vi "clear the mutation history for the classes.vi"(11 "Path":path=path "D:/OneDrive - NI/_WorkingOn/CSM/Communicable-State-Machine/src/user.lib/_NEVSTOP/Communicable State Machine(CSM)/_Support/Priority Queue/Priority Queue.lvclass") -> ()   [LabVIEW 2017]
uses:
  <vilib>/Utility/EditLVLibs/LVClass/Mutation History.ctl
  <vilib>/Utility/EditLVLibs/LVClass/Mutation Record.ctl
  <vilib>/Utility/EditLVLibs/LibVersion.ctl
  <vilib>/Utility/EditLVLibs/Edit LVLibs.lvlib
panel:
  out "Mutation History":T1 {"LabVIEW Version" format="%.0x"}
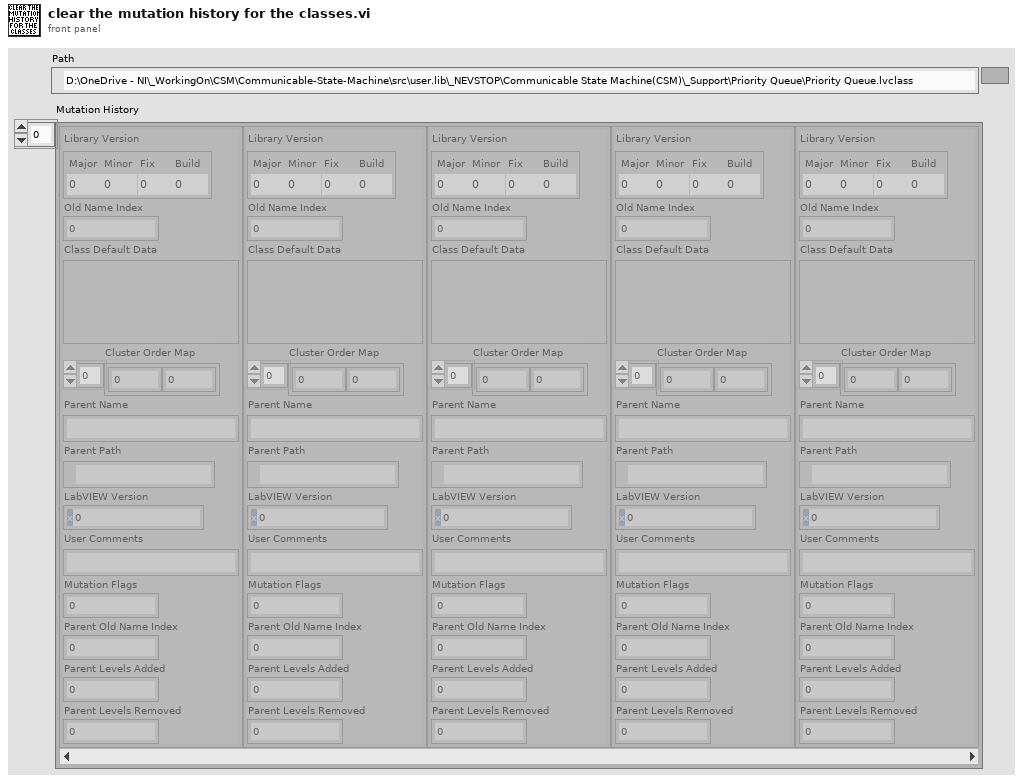
[diagram p1: front panel]
types:
  T1 = typedef "Edit LVLibs.lvlib/Mutation History.ctl" = T2[]
  T2 = typedef "Edit LVLibs.lvlib/Mutation Record.ctl" = cluster{"Library Version":T3, "Old Name Index":u8, "Class Default Data":variant, "Cluster Order Map":u32[], "Parent Name":string, "Parent Path":path, "LabVIEW Version":u32, "User Comments":string, "Mutation Flags":u8, "Parent Old Name Index":u8, "Parent Levels Added":u16, "Parent Levels Removed":u16}
  T3 = typedef "Edit LVLibs.lvlib/LibVersion.ctl" = cluster{"Major":u16, "Minor":u16, "Fix":u16, "Build":u16}
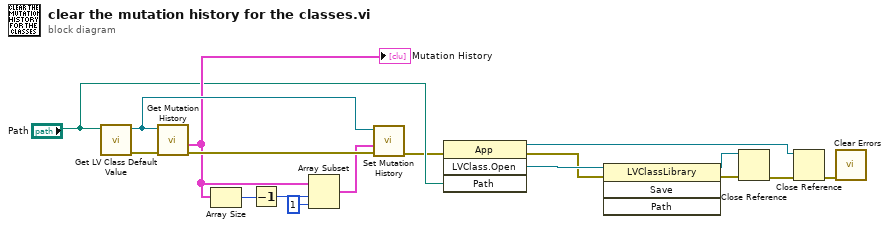
[diagram p0: block diagram]
diagram:
  n1 = call <vilib>:"Get LV Class Default Value.vi"("class path"="Path") -> ("error out"=w16:errorcluster, "object"=w14:refnum<class>)  [unwired: 9 in]
  n2 = call <vilib>:"Get Mutation History.vi"("error in"=w16, "Input object"=w14) -> ("error out"=w17:errorcluster, "Mutation History"=w11:T1)  [unwired: 6 in]
  "Mutation History" <- w11
  n3 = Array Size(array=w11) -> (size(s)=w13:i32)
  n4 = Decrement(x=w13) -> (x-1=w10:i32)
  n5 = Array Subset(array=w11, index=w10, length=1) -> (w15:T1)
  n6 = call <vilib>:"Set Mutation History.vi"("error in"=w17, "Mutation History"=w15, "Input object"=w14) -> ("error out"=w2:errorcluster)  [unwired: 8 in]
  n7 = invoke class="App" method="LVClass.Open"(error in=w2, "Path"="Path") -> (reference out=w3:refnum<vi>, error out=w5:errorcluster, "LVClass.Open"=w9:refnum<vi>)  [unwired: 2 in, 1 out]
  n8 = invoke class="LVClassLibrary" method="Save"(reference=w9, error in=w5) -> (reference out=w7:refnum<vi>, error out=w8:errorcluster)  [unwired: 2 in, 2 out]
  n9 = Close Reference(reference=w7, error in (no error)=w8) -> (error out=w4:errorcluster)
  n10 = Close Reference(reference=w3, error in (no error)=w4) -> (error out=w1:errorcluster)
  n11 = call <vilib>:"Clear Errors.vi"("error in (no error)"=w1) -> ()  [unwired: 5 in, 2 out]
